vi "振动判定nvh.vi"(7 "Result":refnum<vi>, 9 "振动判定":T1, 10 "振动判定范围":T2, 11 "FFT":cluster{"f0":dbl, "df":dbl, "magnitude":dbl[]}[](graph)) -> (0 "判定项长度":i32, 1 "Limit Specifications":cluster{"x0":dbl, "dx":dbl, "Y":dbl[]}[][](array[cluster]), 2 "FFT 2":cluster{"f0":dbl, "df":dbl, "magnitude":dbl[]}[](graph), 3 "OK？":bool)   [LabVIEW 2020]
uses:
  Global_Variable/Global.vi
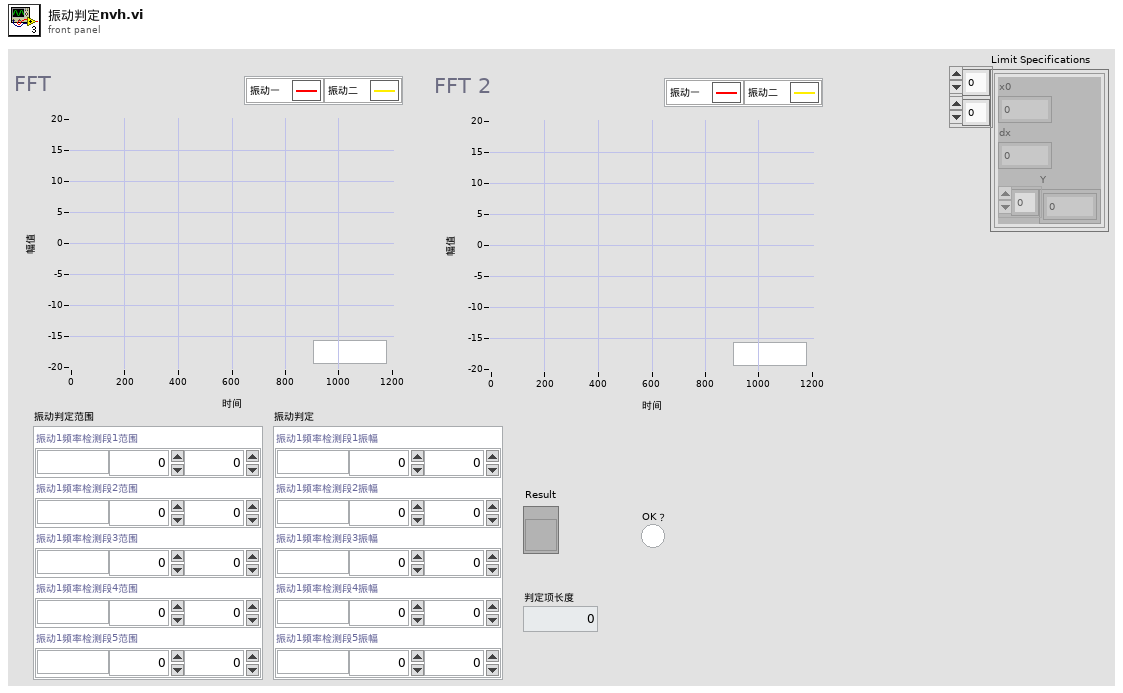
[diagram p1: front panel]
types:
  T1 = cluster{"振动1频率检测段1振幅":cluster{"单位":string, "下限":dbl, "上限":dbl}, "振动1频率检测段2振幅":cluster{"单位":string, "下限":dbl, "上限":dbl}, "振动1频率检测段3振幅":cluster{"单位":string, "下限":dbl, "上限":dbl}, "振动1频率检测段4振幅":cluster{"单位":string, "下限":dbl, "上限":dbl}, "振动1频率检测段5振幅":cluster{"单位":string, "下限":dbl, "上限":dbl}}
  T2 = cluster{"振动1频率检测段1范围":cluster{"单位":string, "下限":dbl, "上限":dbl}, "振动1频率检测段2范围":cluster{"单位":string, "下限":dbl, "上限":dbl}, "振动1频率检测段3范围":cluster{"单位":string, "下限":dbl, "上限":dbl}, "振动1频率检测段4范围":cluster{"单位":string, "下限":dbl, "上限":dbl}, "振动1频率检测段5范围":cluster{"单位":string, "下限":dbl, "上限":dbl}}
  T3 = typedef "svc_Spectrum Info.ctl" = cluster{"channel name":string, "description":string, "x-axis units":T4, "spectral info":cluster{"spectrum type":T5, "linear/dB":enum16{"linear", "dB"}, "window":u16, "window size":i32, "FFT size":i32}, "engineering units":T6, "custom label":string, "dB reference [EU]":dbl, "peak units":enum16{"rms", "peak", "peak-peak"}, "weighting filter":T7, "spectral density?":bool, "unit label":string, "spectrum skewed?":bool, "complimentary spectrum units":T8}
  T4 = typedef "svc_X-Axis Units.ctl" = u16
  T5 = typedef "svc_Spectrum Type.ctl" = enum16{"FFT Spectrum [complex]", "Amplitude [Magnitude]", "Power [Magnitude^2]", "Cross Spectrum [complex]", "Frequency Response [Complex]"}
  T6 = typedef "svc_Engineering Units Text Ring.ctl" = u16
  T7 = typedef "svc_Weighting Filter Text Ring.ctl" = u16
  T8 = typedef "svc_Complimentary Spectrum Units.ctl" = enum16{"none", "radians", "degrees", "cycles", "imaginary"}
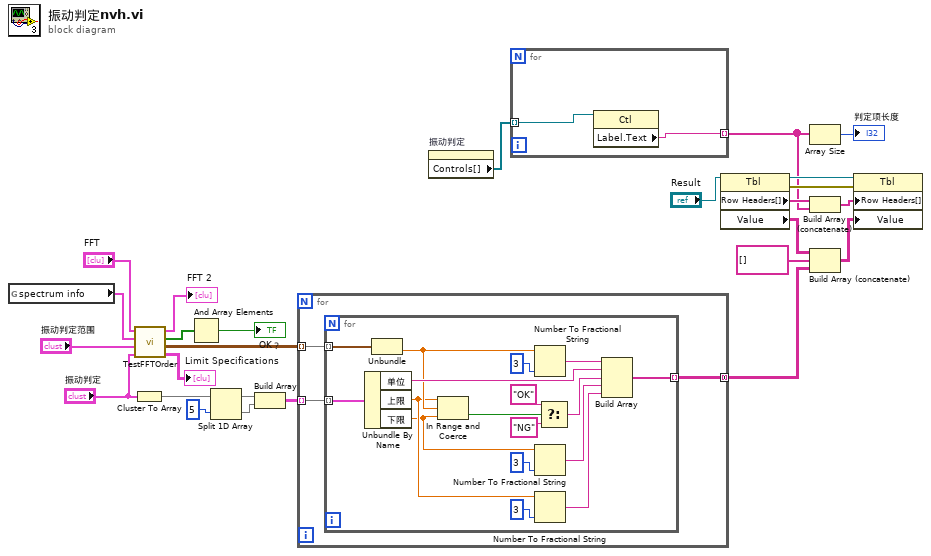
[diagram p0: block diagram]
diagram:
  n1 = global read "Global.vi" "spectrum info"() -> (w25:T3[])
  n2 = Cluster To Array(cluster="振动判定") -> (array=w13:cluster{"单位":string, "下限":dbl, "上限":dbl}[])
  n3 = call "TestFFTOrder.vi"("振动判定"="振动判定", "振动判定范围"="振动判定范围", "spectrum info"=w25, "FFT 5"="FFT") -> ("Limit Specifications"=→"Limit Specifications":cluster{"x0":dbl, "dx":dbl, "Y":dbl[]}[][], "数组"=w18:cluster{"freq.":dbl, "dB":dbl}[][], "Test Result"=w7:bool[], "FFT 2"=→"FFT 2":cluster{"x0":dbl, "dx":dbl, "Y":dbl[]}[])  [unwired: 4 in]
  n4 = And Array Elements(Boolean array=w7) -> (logical AND=→"OK？":bool)
  n5 = Split 1D Array(array=w13, index=5 ("索引")) -> (first subarray=w12:cluster{"单位":string, "下限":dbl, "上限":dbl}[], second subarray=w11:cluster{"单位":string, "下限":dbl, "上限":dbl}[])
  n6 = Build Array(w12, w11) -> (w10:cluster{"单位":string, "下限":dbl, "上限":dbl}[][])
  n7 = for {
    tunnel: w18 -> [w29] mode=indexing
    tunnel: [w27] -> w6 mode=concatenating
    tunnel: w10 -> [w28] mode=indexing
    n8 = for {
      tunnel: w29 -> [w46] mode=indexing
      tunnel: w28 -> [w44] mode=indexing
      tunnel: [w39] -> w27 mode=indexing
      n9 = Unbundle By Name(w44) -> ("单位"=w41:string, "上限"=w33:dbl, "下限"=w32:dbl)
      n10 = Unbundle(w46) -> ("dB"=w37:dbl)  [unwired: 1 out]
      n11 = In Range and Coerce(upper limit=w33, x=w37, lower limit=w32) -> (In Range?=w36:bool)  [unwired: 1 out]
      n12 = Number To Fractional String(number=w37, precision (6)=i16 3 ("精度(6)")) -> (F-format string=w40:string)  [unwired: 2 in]
      n13 = Number To Fractional String(number=w32, precision (6)=i16 3 ("精度(6)")) -> (F-format string=w31:string)  [unwired: 2 in]
      n14 = Number To Fractional String(number=w33, precision (6)=i16 3 ("精度(6)")) -> (F-format string=w30:string)  [unwired: 2 in]
      n15 = Select(t="OK", s=w36, f="NG") -> (s? t:f=w42:string)
      n16 = Build Array(w40, w41, w42, w31, w30) -> (w39:string[])
    }
  }
  n17 = property on="振动判定" class="Clust (严格)"() -> ("Controls[]"=w19:refnum<vi>[])  [unwired: 2 in, 2 out]
  n18 = for {
    tunnel: w19 -> [w48] mode=indexing
    tunnel: [w47] -> w5 mode=indexing
    n19 = property class="Ctl"(reference=w48) -> ("Label.Text"=w47:string)  [unwired: 1 in, 2 out]
  }
  n20 = property class="Tbl"(reference="Result") -> (reference out=w23:refnum<vi>, error out=w24:errorcluster, "Row Headers[]"=w20:string[], "Value"=w17:string[][])  [unwired: 1 in]
  n21 = Array Size(array=w5) -> (size(s)=→"判定项长度":i32)
  n22 = Build Array (concatenate)(w20, w5) -> (w22:string[])
  n23 = Build Array (concatenate)(w17, string[] [] ("数组"), w6) -> (w16:string[][])
  n24 = property class="Tbl"(reference=w23, error in=w24, "Row Headers[]"=w22, "Value"=w16) -> ()  [unwired: 2 out]
